vi "getWaypoints.vi"(8 "Error In":errorcluster, 11 "GenericMission in":refnum<class "GenericMission.lvclass">) -> (0 "Error Out":errorcluster, 2 "Waypoint Array":refnum<class "Waypoint.lvclass">[](array[class]), 3 "GenericMission out":refnum<class "GenericMission.lvclass">)   [LabVIEW 2013, in "GenericMission.lvclass"]
doc: "Returns the array of waypoints required to complete the mission\n\n\n-Kaitlin Gallagher"
uses:
  GenericMission.lvclass
  Waypoint/Waypoint.lvclass
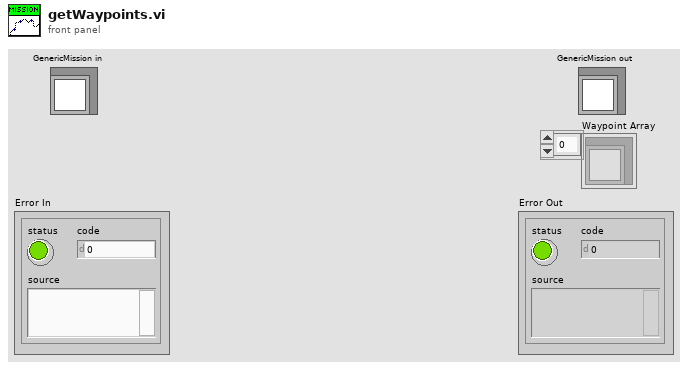
[diagram p1: front panel]
types:
  T1 = typedef "UTM Location.ctl" = cluster{"UTM Zone":dbl, "Hemisphere":enum16{"North", "South"}, "East":dbl, "North":dbl}
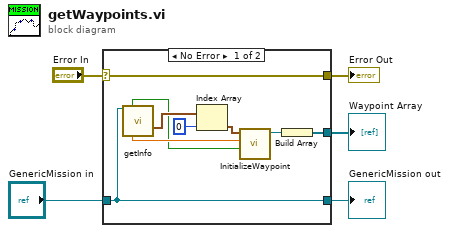
[diagram p0: block diagram]
diagram:
  n1 = case shown="No Error" "Error In" {
    selector: "Error In" -> [w14 w15]
    tunnel: [w14 w15] -> w4
    tunnel: "GenericMission in" -> [w13 w16]
    tunnel: [w13 w16] -> w3
    tunnel: [w7 _] -> w1
    frame No Error {
      n2 = call-dynamic "getInfo.vi"("GenericMission in"=w13) -> ("Done"=w6:bool, "Points of Interest"=w11:T1[], "Tolerance (m)"=w9:dbl)  [unwired: 6 in, 6 out]
      n3 = Index Array(array=w11, index=0) -> (element=w10:T1)
      n4 = call "InitializeWaypoint.vi"("Done?"=w6, "Tolerance (meters?)"=w9, "Coords"=w10) -> ("Waypoint Out"=w8:refnum<class "Waypoint.lvclass">)  [unwired: 8 in]
      n5 = Build Array(w8) -> (w7:refnum<class "Waypoint.lvclass">[])
    }
    frame Error {
    }
  }
  "Error Out" <- w4
  "GenericMission out" <- w3
  "Waypoint Array" <- w1
